vi "Handle IDN.vi"(8 "error in (no error)":errorcluster, 10 "Command":variant, 11 "Instrument in":refnum<class "Instrument.lvclass">) -> (0 "error out":errorcluster, 2 "Variant":variant, 3 "Instrument out":refnum<class "Instrument.lvclass">)   [LabVIEW 2019, in "Instrument.lvclass"]
uses:
  Instrument.lvclass
  Typedefs/Instrument.Commands--Enum.ctl
  Typedefs/PrivateEvents--Instrument.DataToLog.ctl
  Help/Help.lvclass
panel:
  out "<JSON>":string
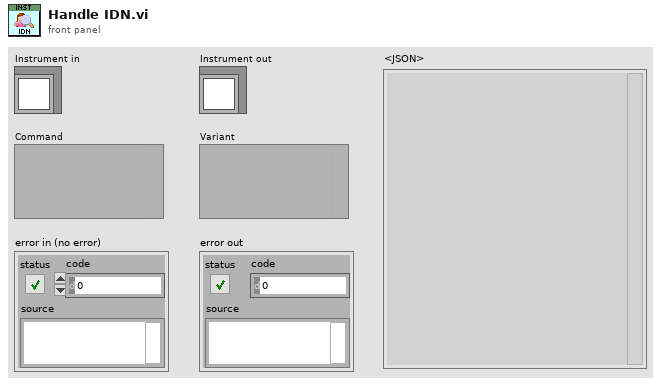
[diagram p1: front panel]
types:
  T1 = typedef "Instrument.lvclass/PrivateEvents--Instrument.DataToLog.ctl" = cluster{"Path(s)":string, "Data":variant}
  T2 = typedef "Instrument.lvclass/Instrument.Commands--Enum.ctl" = enum16{"ACK", "HELP", "IDN", "setConfiguration", "setLogData", "getAll", "getAllData"}
  T3 = cluster{"number1":dbl, "number2":dbl, "string1":string}
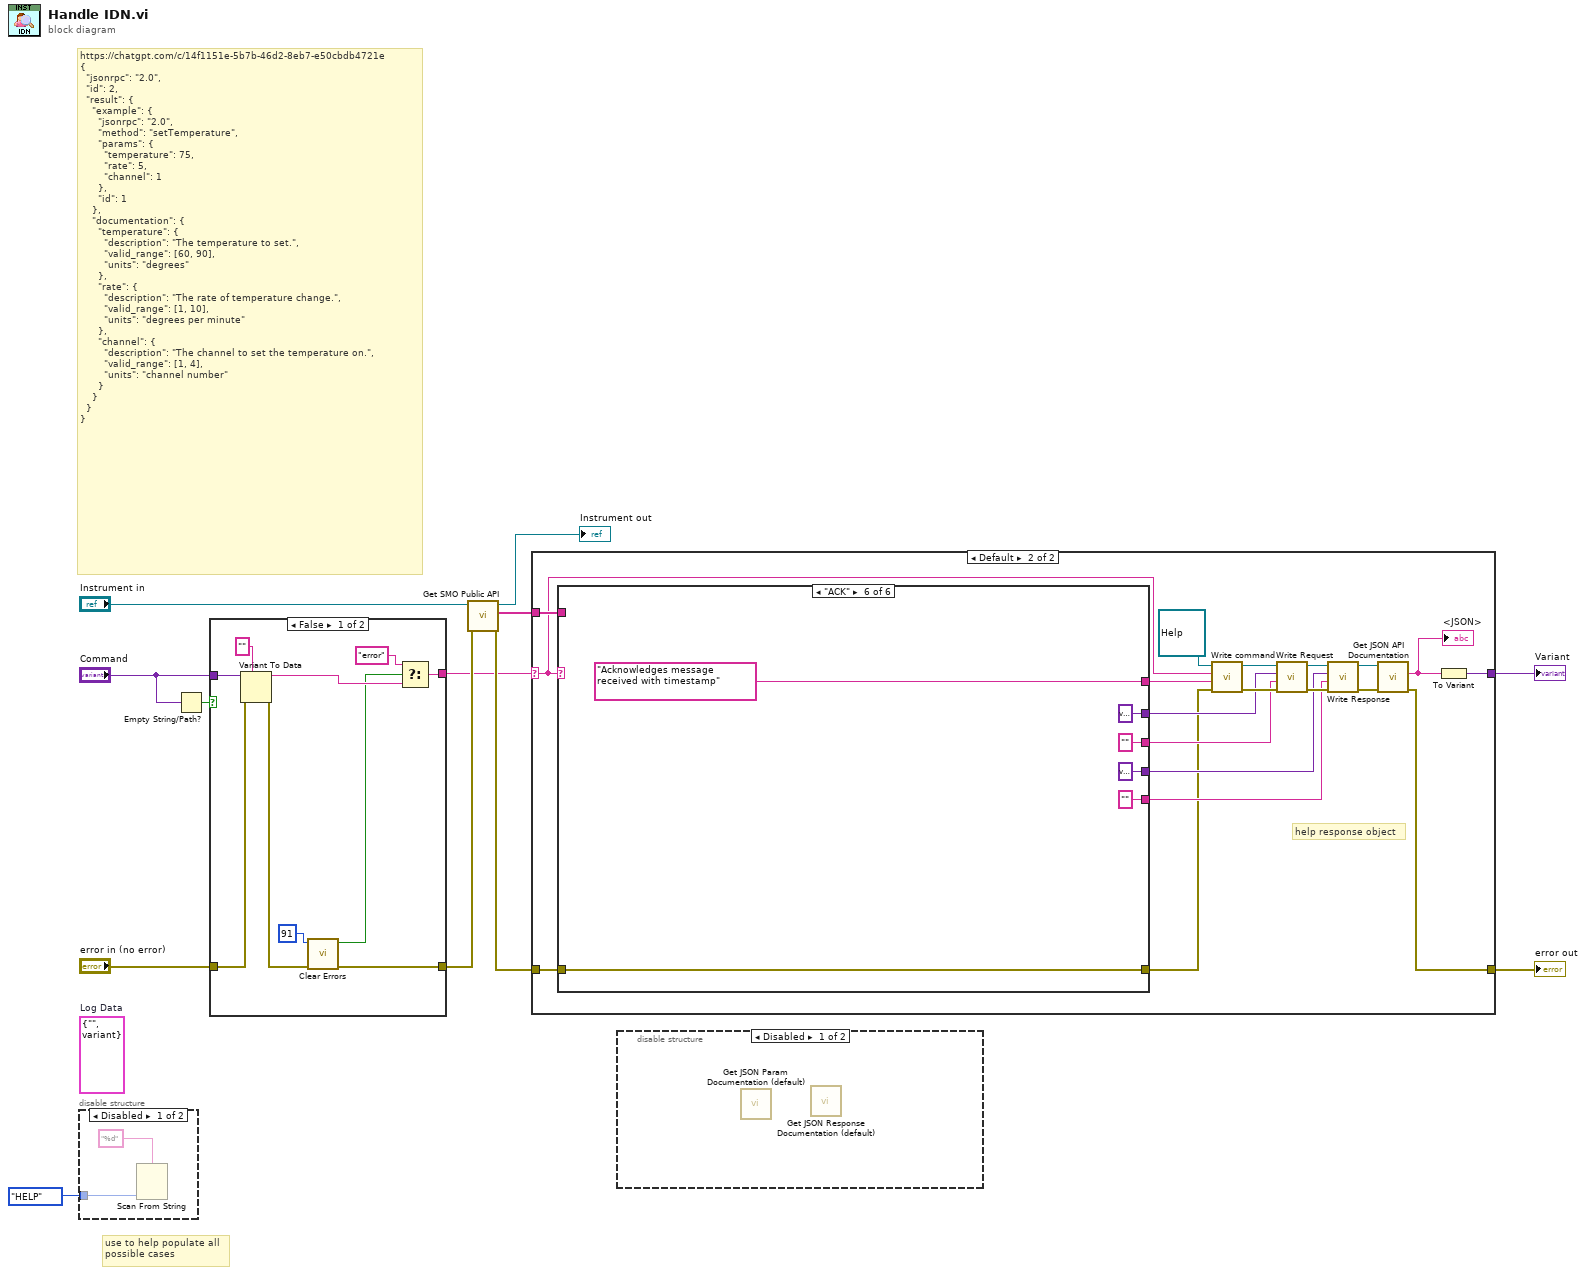
[diagram p0: block diagram]
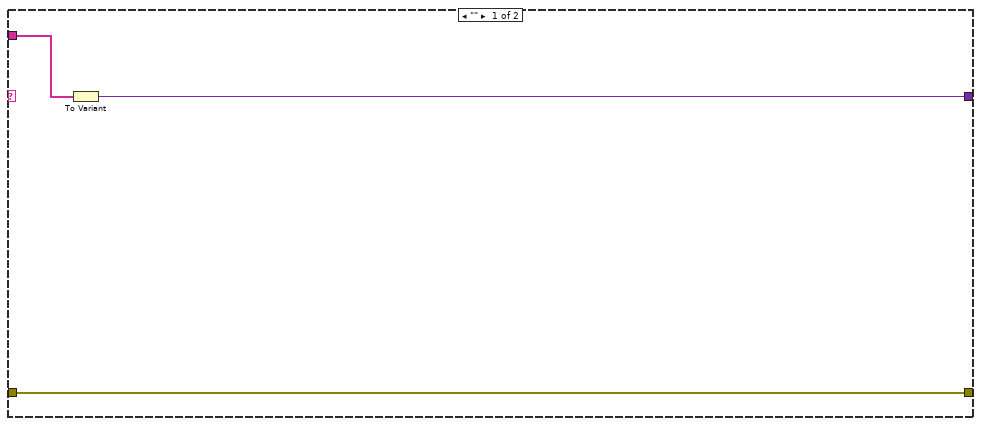
[diagram p2: hidden frame]
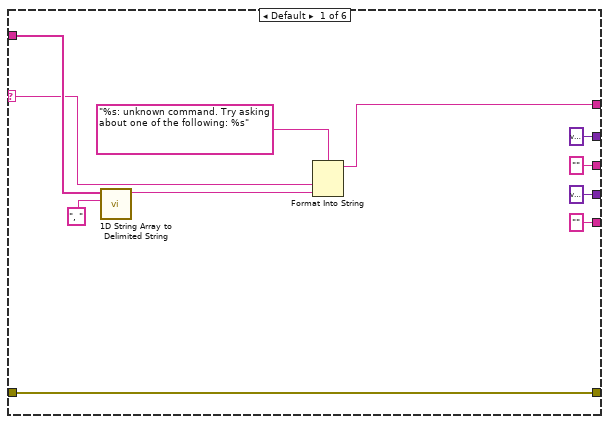
[diagram p3: hidden frame]
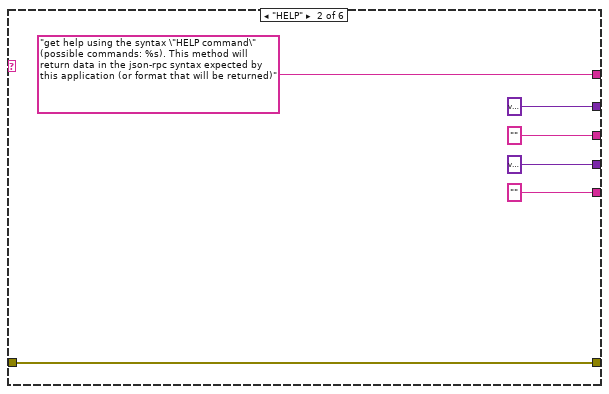
[diagram p4: hidden frame]
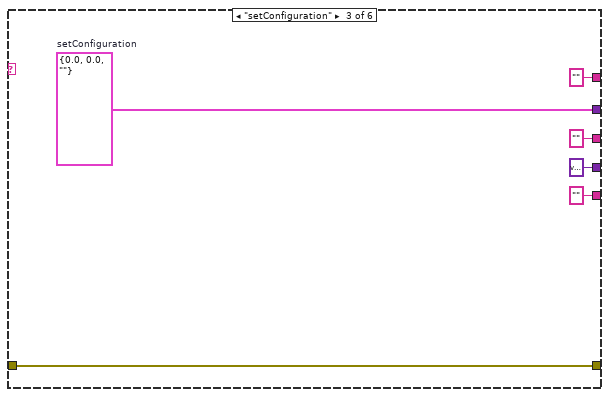
[diagram p5: hidden frame]
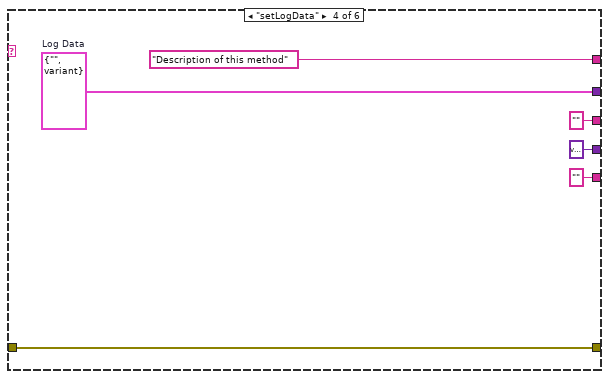
[diagram p6: hidden frame]
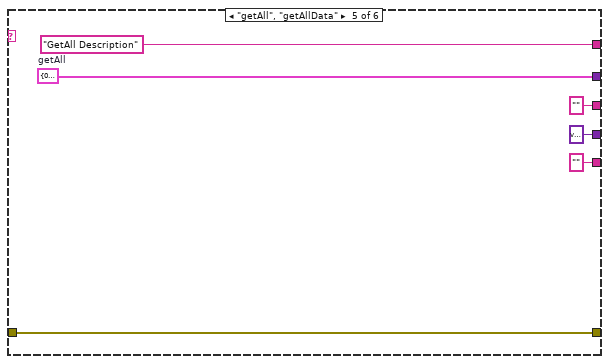
[diagram p7: hidden frame]
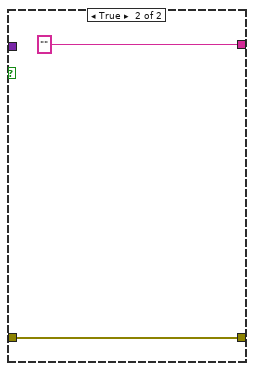
[diagram p8: hidden frame]
diagram:
  (unwired) T1 {"Path(s)"="", "Data"=variant}  # Log Data
  # "https://chatgpt.com/c/14f1151e-5b7b-46d2-8eb7-e50cbdb4721e\n{\n  \"jsonrpc\": \"2.0\",\n  \"id\": 2,\n  \"result\": {\n    \"example\": {\n      \"jsonrpc\": \"2.0\",\n      \"method\": \"setTemperature\",\n      \"params\": {\n        \"temperature\": 75,\n        \"rate\": 5,\n        \"channel\": 1\n      },\n      \"id\": 1\n    },\n    \"documentation\": {\n      \"temperature\": {\n        \"description\": \"The temperature to set.\",\n        \"valid_range\": [60, 90],\n        \"units\": \"degrees\"\n      },\n      \"rate\": {\n        \"description\": \"The rate of temperature change.\",\n        \"valid_range\": [1, 10],\n        \"units\": \"degrees per minute\"\n      },\n      \"channel\": {\n        \"description\": \"The channel to set the temperature on.\",\n        \"valid_range\": [1, 4],\n        \"units\": \"channel number\"\n      }\n    }\n  }\n}"
  # "use to help populate all\npossible cases"
  n1 = disable-structure shown="Disabled" {
    disable-tunnel: Instrument.Commands--Enum."HELP" ("Commands") -> [w14 _]
    frame Disabled {
      n2 = Scan From String(format string="%d", default 1=w14) -> (input string=w15:string)  [unwired: 3 in, 3 out]
    }
    frame Enabled {
    }
  }
  n3 = Empty String/Path?(string/path="Command") -> (empty?=w11:bool)
  n4 = case shown="False" w11 {
    tunnel: "error in (no error)" -> [w25 w27]
    tunnel: [w19 ""] -> w4
    tunnel: [w21 w27] -> w6
    tunnel: "Command" -> [w23 _]
    frame False {
      n5 = Variant To Data(error in=w25, type="", Variant=w23) -> (data=w20:string, error out=w22:errorcluster)
      n6 = call <vilib>:"Clear Errors.vi"("error in (no error)"=w22, "specific error code to clear (0: all)"=91) -> ("error out"=w21:errorcluster, "specific error cleared?"=w16:bool)  [unwired: 4 in]
      n7 = Select(t="error", s=w16, f=w20) -> (s? t:f=w19:string)
    }
    frame True {
    }
  }
  n8 = call-dynamic "Get SMO Public API.vi"("error in (no error)"=w6, "Instrument in"="Instrument in") -> ("error out"=w5:errorcluster, "commands"=w9:string[], "Instrument out"=→"Instrument out":refnum<class "Instrument.lvclass">)  [unwired: 7 in]
  n9 = case shown="Default" w4 {
    selector: w4 -> [_ w34]
    tunnel: w9 -> [w30 w49]
    tunnel: w5 -> [w28 w48]
    tunnel: [w29 w33] -> w2
    tunnel: [w28 w35] -> w1
    frame "" {
      n10 = To Variant(anything=w30) -> (Variant=w29:variant)
    }
    frame Default {
      # "help response object"
      n11 = case shown="\"ACK\"" w34 {
        selector: w34 -> [w51 _ _ _ _ _]
        tunnel: w48 -> [w58 w66 w72 w75 w83 w90]
        tunnel: [w58 w66 w72 w75 w83 w90] -> w31
        tunnel: w49 -> [w57 _ _ _ _ _]
        tunnel: [w56 "get help using the syntax \"HELP command\" (possible commands: %s). This method will return data in the json-rpc syntax expected by this application (or format that will be returned)" "" "Description of this method" ("description") "GetAll Description" "Acknowledges message received with timestamp"] -> w41
        tunnel: [variant ("request cluster") variant ("request cluster") w71 w73 w79 variant ("request cluster")] -> w40
        tunnel: ["" ("<JSON> request documentation") "" ("<JSON> request documentation") "" ("<JSON> request documentation") "" ("<JSON> request documentation") "" ("<JSON> request documentation") "" ("<JSON> request documentation")] -> w39
        tunnel: ["" ("<JSON> response documentation") "" ("<JSON> response documentation") "" ("<JSON> response documentation") "" ("<JSON> response documentation") "" ("<JSON> response documentation") "" ("<JSON> response documentation")] -> w38
        tunnel: [variant ("response cluster") variant ("response cluster") variant ("response cluster") variant ("response cluster") variant ("response cluster") variant ("response cluster")] -> w37
        frame Default {
          n12 = call <vilib>:"1D String Array to Delimited String.vi"("delimiter"=", ", "string array"=w57) -> ("delimited string"=w59:string)  [unwired: 9 in]
          n13 = Format Into String(format string="%s: unknown command. Try asking about one of the following: %s", w51, w59) -> (resulting string=w56:string)  [unwired: 2 in, 1 out]
        }
        frame "HELP" {
        }
        frame "setConfiguration" {
          w71 = T3 {"number1"=0.0, "number2"=0.0, "string1"=""}  # setConfiguration
        }
        frame "setLogData" {
          w73 = T1 {"Path(s)"="", "Data"=variant}  # Log Data
        }
        frame "getAll", "getAllData" {
          w79 = T3 {"number1"=0.0, "number2"=0.0, "string1"=""}  # getAll
        }
        frame "ACK" {
        }
      }
      n14 = call "Write command.vi"("error in (no error)"=w31, "command description"=w41, "command"=w34, "Help in"=refnum<class "Help.lvclass"> refnum) -> ("error out"=w47:errorcluster, "Help out"=w42:refnum<class "Help.lvclass">)  [unwired: 6 in]
      n15 = call "Write Request.vi"("error in (no error)"=w47, "<JSON> request documentation"=w39, "request cluster"=w40, "Help in"=w42) -> ("error out"=w46:errorcluster, "Help out"=w43:refnum<class "Help.lvclass">)  [unwired: 6 in]
      n16 = call "Write Response.vi"("error in (no error)"=w46, "<JSON> response documentation"=w38, "response cluster"=w37, "Help in"=w43) -> ("error out"=w45:errorcluster, "Help out"=w44:refnum<class "Help.lvclass">)  [unwired: 6 in]
      n17 = call "Get JSON API Documentation.vi"("error in (no error)"=w45, "Help"=w44) -> ("error out"=w35:errorcluster, "<JSON> API doc"=w36:string)  [unwired: 7 in, 1 out]
      "<JSON>" <- w36
      n18 = To Variant(anything=w36) -> (Variant=w33:variant)
    }
  }
  "Variant" <- w2
  "error out" <- w1
  n19 = disable-structure shown="Disabled" {
    frame Disabled {
      n20 = call "Get JSON Param Documentation (default).vi"() -> ()  [unwired: 10 in, 2 out]
      n21 = call "Get JSON Response Documentation (default).vi"() -> ()  [unwired: 10 in, 2 out]
    }
    frame Enabled {
    }
  }
